vi "rsscope_core_global.vi"() -> ()   [LabVIEW 2018] (continued)
of the modulation signal for the FM modulation types.\n\nAvailable Repeated Capabilities:\nWaveformGenerator: WG1, WG2\r\n\nRemote-control command(s):\nWGENerator<m>:MODulation:FM[:FUNCtion]"}, {"Level"=5, "Class Only"=FALSE, "Identifier"="RSSCOPE_ATTR_WAVEFORM_GENERATOR_FM_MODULATION_FREQUENCY", "Descriptive Name"="Waveform Generator FM Modulation Frequency", "Data Type"=1, "Command"="WGEN{WaveformGenerator}:MOD:FM:FREQ", "Access"=2, "Range Table"="RsScope_rngWaveformGeneratorModulationFrequency", "Read Callback"="", "Write Callback"="", "Supported Models"="", "Instrument Options"="B6", "Flags"=0, "Help"="Sets the frequency of the modulation waveform for frequency modulation.\n\nAvailable Repeated Capabilities:\nWaveformGenerator: WG1, WG2\r\n\nRemote-control command(s):\nWGENerator<m>:MODulation:FM:FREQuency"}, {"Level"=5, "Class Only"=FALSE, "Identifier"="RSSCOPE_ATTR_WAVEFORM_GENERATOR_FM_MODULATION_FREQUENCY_DEVIATION", "Descriptive Name"="Waveform Generator FM Modulation Frequency Deviation", "Data Type"=1, "Command"="WGEN{WaveformGenerator}:MOD:FM:DEV", "Access"=2, "Range Table"="RsScope_rngWaveformGeneratorFMModulationFrequencyDeviation", "Read Callback"="", "Write Callback"="", "Supported Models"="", "Instrument Options"="B6", "Flags"=0, "Help"="Sets the frequency deviation, the maximum difference between and FM modulated signal and the carrier signal.\n\nAvailable Repeated Capabilities:\nWaveformGenerator: WG1, WG2\r\n\nRemote-control command(s):\nWGENerator<m>:MODulation:FM:DEViation"}, {"Level"=5, "Class Only"=FALSE, "Identifier"="RSSCOPE_ATTR_WAVEFORM_GENERATOR_FM_MODULATION_DUTY_CYCLE", "Descriptive Name"="Waveform Generator FM Modulation Duty Cycle", "Data Type"=1, "Command"="WGEN{WaveformGenerator}:MOD:FM:DCYC", "Access"=2, "Range Table"="RsScope_rngWaveformGeneratorModulationDutyCycle", "Read Callback"="", "Write Callback"="", "Supported Models"="", "Instrument Options"="B6", "Flags"=0, "Help"="Sets the duty cycle of a square waveform for frequency modulation.\n\nAvailable Repeated Capabilities:\nWaveformGenerator: WG1, WG2\r\n\nRemote-control command(s):\nWGENerator<m>:MODulation:FM:DCYCle"}, {"Level"=5, "Class Only"=FALSE, "Identifier"="RSSCOPE_ATTR_WAVEFORM_GENERATOR_FM_MODULATION_SYMMETRY", "Descriptive Name"="Waveform Generator FM Modulation Symmetry", "Data Type"=1, "Command"="WGEN{WaveformGenerator}:MOD:FM:SYMM", "Access"=2, "Range Table"="RsScope_rngPercent", "Read Callback"="", "Write Callback"="", "Supported Models"="", "Instrument Options"="B6", "Flags"=0, "Help"="Sets the symmetry, the percentage of time the ramp modulation waveform is rising, for frequency modulation.\n\nAvailable Repeated Capabilities:\nWaveformGenerator: WG1, WG2\r\n\nRemote-control command(s):\nWGENerator<m>:MODulation:FM:SYMMetry"}, {"Level"=4, "Class Only"=TRUE, "Identifier"="", "Descriptive Name"="PWM", "Data Type"=0, "Command"="", "Access"=0, "Range Table"="", "Read Callback"="", "Write Callback"="", "Supported Models"="", "Instrument Options"="", "Flags"=0, "Help"="For pulse width modulation (PWM), the time for which the signal is in a high state is varied according to the modulation signal."}, {"Level"=5, "Class Only"=FALSE, "Identifier"="RSSCOPE_ATTR_WAVEFORM_GENERATOR_PWM_MODULATION_SIGNAL", "Descriptive Name"="Waveform Generator PWM Modulation Signal", "Data Type"=0, "Command"="WGEN{WaveformGenerator}:MOD:PWM", "Access"=2, "Range Table"="RsScope_rngWaveformGeneratorModulationSignal", "Read Callback"="", "Write Callback"="", "Supported Models"="", "Instrument Options"="B6", "Flags"=0, "Help"="Selects the type of the modulation signal for the PWM modulation types.\n\nAvailable Repeated Capabilities:\nWaveformGenerator: WG1, WG2\r\n\nRemote-control command(s):\nWGENerator<m>:MODulation:PWM[:FUNCtion]"}, {"Level"=5, "Class Only"=FALSE, "Identifier"="RSSCOPE_ATTR_WAVEFORM_GENERATOR_PWM_MODULATION_FREQUENCY", "Descriptive Name"="Waveform Generator PWM Modulation Frequency", "Data Type"=1, "Command"="WGEN{WaveformGenerator}:MOD:PWM:FREQ", "Access"=2, "Range Table"="RsScope_rngWaveformGeneratorModulationFrequency", "Read Callback"="", "Write Callback"="", "Supported Models"="", "Instrument Options"="B6", "Flags"=0, "Help"="Sets the type of the modulation signal for the pulse width modulation.\n\nAvailable Repeated Capabilities:\nWaveformGenerator: WG1, WG2\r\n\nRemote-control command(s):\nWGENerator<m>:MODulation:PWM:FREQuency"}, {"Level"=5, "Class Only"=FALSE, "Identifier"="RSSCOPE_ATTR_WAVEFORM_GENERATOR_PWM_MODULATION_DEPTH", "Descriptive Name"="Waveform Generator PWM Modulation Depth", "Data Type"=1, "Command"="WGEN{WaveformGenerator}:MOD:PWM:DEPT", "Access"=2, "Range Table"="RsScope_rngPercent", "Read Callback"="", "Write Callback"="", "Supported Models"="", "Instrument Options"="B6", "Flags"=0, "Help"="Sets the modulation depth for pulse width modulation.\n\nAvailable Repeated Capabilities:\nWaveformGenerator: WG1, WG2\r\n\nRemote-control command(s):\nWGENerator<m>:MODulation:PWM:DEPTh"}, {"Level"=5, "Class Only"=FALSE, "Identifier"="RSSCOPE_ATTR_WAVEFORM_GENERATOR_PWM_MODULATION_DUTY_CYCLE", "Descriptive Name"="Waveform Generator PWM Modulation Duty Cycle", "Data Type"=1, "Command"="WGEN{WaveformGenerator}:MOD:PWM:DCYC", "Access"=2, "Range Table"="RsScope_rngWaveformGeneratorModulationDutyCycle", "Read Callback"="", "Write Callback"="", "Supported Models"="", "Instrument Options"="B6", "Flags"=0, "Help"="Sets the duty cycle of a square waveform for pulse width modulation.\n\nAvailable Repeated Capabilities:\nWaveformGenerator: WG1, WG2\r\n\nRemote-control command(s):\nWGENerator<m>:MODulation:PWM:DCYCle"}, {"Level"=5, "Class Only"=FALSE, "Identifier"="RSSCOPE_ATTR_WAVEFORM_GENERATOR_PWM_MODULATION_SYMMETRY", "Descriptive Name"="Waveform Generator PWM Modulation Symmetry", "Data Type"=1, "Command"="WGEN{WaveformGenerator}:MOD:PWM:SYMM", "Access"=2, "Range Table"="RsScope_rngPercent", "Read Callback"="", "Write Callback"="", "Supported Models"="", "Instrument Options"="B6", "Flags"=0, "Help"="Sets the symmetry, the percentage of time the ramp modulation waveform is rising, for pulse width modulation.\n\nAvailable Repeated Capabilities:\nWaveformGenerator: WG1, WG2\r\n\nRemote-control command(s):\nWGENerator<m>:MODulation:PWM:SYMMetry"}, {"Level"=4, "Class Only"=TRUE, "Identifier"="", "Descriptive Name"="FSK", "Data Type"=0, "Command"="", "Access"=0, "Range Table"="", "Read Callback"="", "Write Callback"="", "Supported Models"="", "Instrument Options"="", "Flags"=0, "Help"="For frequency shift keying (FSK) modulation, the signal switches between Frequency 1 and Frequency 2 at a Hop rate."}, {"Level"=5, "Class Only"=FALSE, "Identifier"="RSSCOPE_ATTR_WAVEFORM_GENERATOR_FSK_MODULATION_FREQUENCY_1", "Descriptive Name"="Waveform Generator FSK Modulation Frequency 1", "Data Type"=1, "Command"="WGEN{WaveformGenerator}:MOD:FSK:FONE", "Access"=2, "Range Table"="RsScope_rngWaveformGeneratorFrequency", "Read Callback"="", "Write Callback"="", "Supported Models"="", "Instrument Options"="B6", "Flags"=0, "Help"="Sets the frequency of the carrier waveform.\n\nAvailable Repeated Capabilities:\nWaveformGenerator: WG1, WG2\r\n\nRemote-control command(s):\nWGENerator<m>:MODulation:FSK:FONE"}, {"Level"=5, "Class Only"=FALSE, "Identifier"="RSSCOPE_ATTR_WAVEFORM_GENERATOR_FSK_MODULATION_FREQUENCY_2", "Descriptive Name"="Waveform Generator FSK Modulation Frequency 2", "Data Type"=1, "Command"="WGEN{WaveformGenerator}:MOD:FSK:FTWO", "Access"=2, "Range Table"="RsScope_rngWaveformGeneratorFrequency", "Read Callback"="", "Write Callback"="", "Supported Models"="", "Instrument Options"="B6", "Flags"=0, "Help"="Sets the frequency of the modulated waveform.\n\nAvailable Repeated Capabilities:\nWaveformGenerator: WG1, WG2\r\n\nRemote-control command(s):\nWGENerator<m>:MODulation:FSK:FTWO"}, {"Level"=5, "Class Only"=FALSE, "Identifier"="RSSCOPE_ATTR_WAVEFORM_GENERATOR_FSK_MODULATION_HOP_RATE", "Descriptive Name"="Waveform Generator FSK Modulation Hop Rate", "Data Type"=1, "Command"="WGEN{WaveformGenerator}:MOD:FSK", "Access"=2, "Range Table"="RsScope_rngWaveformGeneratorFSKModulationHopRate", "Read Callback"="", "Write Callback"="", "Supported Models"="", "Instrument Options"="B6", "Flags"=0, "Help"="Sets the hop rate, the time before a switch from the carrier frequency and the modulation frequency.\n\nAvailable Repeated Capabilities:\nWaveformGenerator: WG1, WG2\r\n\nRemote-control command(s):\nWGENerator<m>:MODulation:FSK[:RATE]"}, {"Level"=3, "Class Only"=TRUE, "Identifier"="", "Descriptive Name"="Sweep", "Data Type"=0, "Command"="", "Access"=0, "Range Table"="", "Read Callback"="", "Write Callback"="", "Supported Models"="", "Instrument Options"="", "Flags"=0, "Help"="In the sweep mode, the R&S RTO generates a signal whose frequency gradually changes from the Start frequency to the Stop freuqency for a certain Sweep time."}, {"Level"=4, "Class Only"=FALSE, "Identifier"="RSSCOPE_ATTR_WAVEFORM_GENERATOR_SWEEP_START_FREQUENCY", "Descriptive Name"="Waveform Generator Sweep Start Frequency", "Data Type"=1, "Command"="WGEN{WaveformGenerator}:SWE:FST", "Access"=2, "Range Table"="RsScope_rngWaveformGeneratorFrequency", "Read Callback"="", "Write Callback"="", "Supported Models"="", "Instrument Options"="B6", "Flags"=0, "Help"="Sets the start frequency of the sweep range.\n\nAvailable Repeated Capabilities:\nWaveformGenerator: WG1, WG2\r\n\nRemote-control command(s):\nWGENerator<m>:SWEep:FSTart"}, {"Level"=4, "Class Only"=FALSE, "Identifier"="RSSCOPE_ATTR_WAVEFORM_GENERATOR_SWEEP_STOP_FREQUENCY", "Descriptive Name"="Waveform Generator Sweep Stop Frequency", "Data Type"=1, "Command"="WGEN{WaveformGenerator}:SWE", "Access"=2, "Range Table"="RsScope_rngWaveformGeneratorFrequency", "Read Callback"="", "Write Callback"="", "Supported Models"="", "Instrument Options"="B6", "Flags"=0, "Help"="Sets the stop frequency of the sweep range.\n\nAvailable Repeated Capabilities:\nWaveformGenerator: WG1, WG2\r\n\nRemote-control command(s):\nWGENerator<m>:SWEep[:FEND]"}, {"Level"=4, "Class Only"=FALSE, "Identifier"="RSSCOPE_ATTR_WAVEFORM_GENERATOR_SWEEP_TIME", "Descriptive Name"="Waveform Generator Sweep Time", "Data Type"=1, "Command"="WGEN{WaveformGenerator}:SWE:TIME", "Access"=2, "Range Table"="RsScope_rngWaveformGeneratorSweepTime", "Read Callback"="", "Write Callback"="", "Supported Models"="", "Instrument Options"="B6", "Flags"=0, "Help"="Sets the duration of the sweep.\n\nAvailable Repeated Capabilities:\nWaveformGenerator: WG1, WG2\r\n\nRemote-control command(s):\nWGENerator<m>:SWEep:TIME"}, {"Level"=3, "Class Only"=TRUE, "Identifier"="", "Descriptive Name"="Arbitrary", "Data Type"=0, "Command"="", "Access"=0, "Range Table"="", "Read Callback"="", "Write Callback"="", "Supported Models"="", "Instrument Options"="", "Flags"=0, "Help"="The arbitrary waveform generator allows you to output a user-defined waveform for testing your devices. You can output a waveform from a file or from the current R&S RTO reference curve format. Files in *.csv and *.bin formats are supported. This files must follow a defined structure."}, {"Level"=4, "Class Only"=FALSE, "Identifier"="RSSCOPE_ATTR_WAVEFORM_GENERATOR_ARBITRARY_SOURCE", "Descriptive Name"="Waveform Generator Arbitrary Source", "Data Type"=0, "Command"="WGEN{WaveformGenerator}:ARBG", "Access"=2, "Range Table"="RsScope_rngWaveformGeneratorArbitrarySource", "Read Callback"="", "Write Callback"="", "Supported Models"="", "Instrument Options"="B6", "Flags"=0, "Help"="Selects the arbitrary waveform source. You can load an existing file or load the current oscilloscope waveform.\n\nAvailable Repeated Capabilities:\nWaveformGenerator: WG1, WG2\r\n\nRemote-control command(s):\nWGENerator<m>:ARBGen[:SOURce]"}, {"Level"=4, "Class Only"=FALSE, "Identifier"="RSSCOPE_ATTR_WAVEFORM_GENERATOR_ARBITRARY_RUN_MODE", "Descriptive Name"="Waveform Generator Arbitrary Run Mode", "Data Type"=0, "Command"="WGEN{WaveformGenerator}:ARBG:RUNM", "Access"=2, "Range Table"="RsScope_rngWaveformGeneratorRunMode", "Read Callback"="", "Write Callback"="", "Supported Models"="", "Instrument Options"="B6", "Flags"=0, "Help"="Sets the duration for which the signal of the arbitrary generator will be output after the trigger event.\n\nAvailable Repeated Capabilities:\nWaveformGenerator: WG1, WG2\r\n\nRemote-control command(s):\nWGENerator<m>:ARBGen:RUNMode"}, {"Level"=4, "Class Only"=FALSE, "Identifier"="RSSCOPE_ATTR_WAVEFORM_GENERATOR_ARBITRARY_RUN_SINGLE", "Descriptive Name"="Waveform Generator Arbitrary Run Single", "Data Type"=4, "Command"="WGEN{WaveformGenerator}:ARBG:RUNS", "Access"=1, "Range Table"="", "Read Callback"="", "Write Callback"="", "Supported Models"="", "Instrument Options"="", "Flags"=0, "Help"="Executes a single period of the arbitrary signal generator.\n\nAvailable Repeated Capabilities:\nWaveformGenerator: WG1, WG2\r\n\nRemote-control command(s):\nWGENerator<m>:ARBGen:RUNSingle"}, {"Level"=4, "Class Only"=FALSE, "Identifier"="RSSCOPE_ATTR_WAVEFORM_GENERATOR_ARBITRARY_SAMPLE_RATE", "Descriptive Name"="Waveform Generator Arbitrary Sample Rate", "Data Type"=0, "Command"="WGEN{WaveformGenerator}:ARBG:SRAT", "Access"=2, "Range Table"="RsScope_rngWaveformGeneratorArbitrarySampleRate", "Read Callback"="", "Write Callback"="", "Supported Models"="", "Instrument Options"="B6", "Flags"=0, "Help"="Sets the sample rate for the arbitrary waveform.\n\nAvailable Repeated Capabilities:\nWaveformGenerator: WG1, WG2\r\n\nRemote-control command(s):\nWGENerator<m>:ARBGen:SRATe"}, {"Level"=4, "Class Only"=FALSE, "Identifier"="RSSCOPE_ATTR_WAVEFORM_GENERATOR_ARBITRARY_SAMPLES", "Descriptive Name"="Waveform Generator Arbitrary Samples", "Data Type"=0, "Command"="WGEN{WaveformGenerator}:ARBG:SAMP?", "Access"=0, "Range Table"="", "Read Callback"="", "Write Callback"="", "Supported Models"="", "Instrument Options"="B6", "Flags"=0, "Help"="Displays the number of samples in the loaded waveform.\n\nAvailable Repeated Capabilities:\nWaveformGenerator: WG1, WG2\r\n\nRemote-control command(s):\nWGENerator<m>:ARBGen:SAMPles?"}, {"Level"=4, "Class Only"=TRUE, "Identifier"="", "Descriptive Name"="Saved Waveform", "Data Type"=0, "Command"="", "Access"=0, "Range Table"="", "Read Callback"="", "Write Callback"="", "Supported Models"="", "Instrument Options"="", "Flags"=0, "Help"="Configures arbitrary saved waveform."}, {"Level"=5, "Class Only"=FALSE, "Identifier"="RSSCOPE_ATTR_WAVEFORM_GENERATOR_ARBITRARY_FILE_NAME", "Descriptive Name"="Waveform Generator Arbitrary File Name", "Data Type"=2, "Command"="WGEN{WaveformGenerator}:ARBG:NAME", "Access"=2, "Range Table"="", "Read Callback"="", "Write Callback"="", "Supported Models"="", "Instrument Options"="B6", "Flags"=0, "Help"="Sets the file path and the file for an arbitrary waveform.\n\nAvailable Repeated Capabilities:\nWaveformGenerator: WG1, WG2\r\n\nRemote-control command(s):\nWGENerator<m>:ARBGen:NAME"}, {"Level"=5, "Class Only"=FALSE, "Identifier"="RSSCOPE_ATTR_WAVEFORM_GENERATOR_ARBITRARY_OPEN_FILE", "Descriptive Name"="Waveform Generator Arbitrary Open File", "Data Type"=4, "Command"="WGEN{WaveformGenerator}:ARBG:OPEN", "Access"=1, "Range Table"="", "Read Callback"="", "Write Callback"="", "Supported Models"="", "Instrument Options"="B6", "Flags"=0, "Help"="Loads the arbitrary waveform.\n\nAvailable Repeated Capabilities:\nWaveformGenerator: WG1, WG2\r\n\nRemote-control command(s):\nWGENerator<m>:ARBGen:OPEN"}, {"Level"=5, "Class Only"=FALSE, "Identifier"="RSSCOPE_ATTR_WAVEFORM_GENERATOR_ARBITRARY_MULTICHANNEL_FILE_NAME", "Descriptive Name"="Waveform Generator Arbitrary Multichannel File Name", "Data Type"=2, "Command"="WGEN{WaveformGenerator}:ARBG:MULT:NAME", "Access"=2, "Range Table"="", "Read Callback"="", "Write Callback"="", "Supported Models"="", "Instrument Options"="B6", "Flags"=0, "Help"="Defines the path and the multichannel arbitrary waveform file to be imported.\n\nAvailable Repeated Capabilities:\nWaveformGenerator: WG1, WG2\r\n\nRemote-control command(s):\nWGENerator<m>:ARBGen:MULTichannel:NAME"}, {"Level"=5, "Class Only"=FALSE, "Identifier"="RSSCOPE_ATTR_WAVEFORM_GENERATOR_ARBITRARY_MULTICHANNEL_OPEN_FILE", "Descriptive Name"="Waveform Generator Arbitrary Multichannel Open File", "Data Type"=4, "Command"="WGEN{WaveformGenerator}:ARBG:MULT:OPEN", "Access"=1, "Range Table"="", "Read Callback"="", "Write Callback"="", "Supported Models"="", "Instrument Options"="B6", "Flags"=0, "Help"="Loads the arbitrary waveform.\n\nAvailable Repeated Capabilities:\nWaveformGenerator: WG1, WG2\r\n\nRemote-control command(s):\nWGENerator<m>:ARBGen:MULTichannel:OPEN"}, {"Level"=5, "Class Only"=FALSE, "Identifier"="RSSCOPE_ATTR_WAVEFORM_GENERATOR_ARBITRARY_MULTICHANNEL_WAVEFORM", "Descriptive Name"="Waveform Generator Arbitrary Multichannel Waveform", "Data Type"=0, "Command"="WGEN{WaveformGenerator}:ARBG:MULT:IMP", "Access"=2, "Range Table"="RsScope_rngWaveformGeneratorArbitraryMultichannelWaveform", "Read Callback"="", "Write Callback"="", "Supported Models"="", "Instrument Options"="B6", "Flags"=0, "Help"="Assigns a waveform from the multichannel file to the arbitrary waveform generator.\n\nAvailable Repeated Capabilities:\nWaveformGenerator: WG1, WG2\r\n\nRemote-control command(s):\nWGENerator<m>:ARBGen:MULTichannel:IMPort"}, {"Level"=4, "Class Only"=TRUE, "Identifier"="", "Descriptive Name"="Scope Waveform", "Data Type"=0, "Command"="", "Access"=0, "Range Table"="", "Read Callback"="", "Write Callback"="", "Supported Models"="", "Instrument Options"="", "Flags"=0, "Help"="Configures arbitrary scope waveform."}, {"Level"=5, "Class Only"=FALSE, "Identifier"="RSSCOPE_ATTR_WAVEFORM_GENERATOR_ARBITRARY_SCOPE_SOURCE", "Descriptive Name"="Waveform Generator Arbitrary Scope Source", "Data Type"=0, "Command"="WGEN{WaveformGenerator}:ARBG:SEL", "Access"=2, "Range Table"="RsScope_rngWaveformGeneratorArbitraryScopeSource", "Read Callback"="", "Write Callback"="", "Supported Models"="", "Instrument Options"="B6", "Flags"=0, "Help"="Selects the oscilloscope source, from which the arbitrary signal is loaded.\n\nAvailable Repeated Capabilities:\nWaveformGenerator: WG1, WG2\r\n\nRemote-control command(s):\nWGENerator<m>:ARBGen:SELect"}, {"Level"=5, "Class Only"=FALSE, "Identifier"="RSSCOPE_ATTR_WAVEFORM_GENERATOR_ARBITRARY_SCOPE_OPEN", "Descriptive Name"="Waveform Generator Arbitrary Scope Open", "Data Type"=4, "Command"="WGEN{WaveformGenerator}:ARBG:COPY", "Access"=1, "Range Table"="", "Read Callback"="", "Write Callback"="", "Supported Models"="", "Instrument Options"="B6", "Flags"=0, "Help"="Loads the waveform from the selected signal source.\n\nAvailable Repeated Capabilities:\nWaveformGenerator: WG1, WG2\r\n\nRemote-control command(s):\nWGENerator<m>:ARBGen:COPY"}, {"Level"=3, "Class Only"=TRUE, "Identifier"="", "Descriptive Name"="Output", "Data Type"=0, "Command"="", "Access"=0, "Range Table"="", "Read Callback"="", "Write Callback"="", "Supported Models"="", "Instrument Options"="", "Flags"=0, "Help"="Configures the output values of generator."}, {"Level"=4, "Class Only"=FALSE, "Identifier"="RSSCOPE_ATTR_WAVEFORM_GENERATOR_OUTPUT_AMPLITUDE", "Descriptive Name"="Waveform Generator Output Amplitude", "Data Type"=1, "Command"="WGEN{WaveformGenerator}:VOLT", "Access"=2, "Range Table"="RsScope_rngWaveformGeneratorOutputAmplitude", "Read Callback"="", "Write Callback"="", "Supported Models"="", "Instrument Options"="B6", "Flags"=0, "Help"="Sets the amplitude, peak to peak voltage, of the output waveform. This is defined as the voltage difference between the maximum and the minimum voltage levels.\n\nAvailable Repeated Capabilities:\nWaveformGenerator: WG1, WG2\r\n\nRemote-control command(s):\nWGENerator<m>:VOLTage[:VPP]"}, {"Level"=4, "Class Only"=FALSE, "Identifier"="RSSCOPE_ATTR_WAVEFORM_GENERATOR_OUTPUT_OFFSET", "Descriptive Name"="Waveform Generator Output Offset", "Data Type"=1, "Command"="WGEN{WaveformGenerator}:VOLT:OFFS", "Access"=2, "Range Table"="RsScope_rngWaveformGeneratorOutputOffset", "Read Callback"="", "Write Callback"="", "Supported Models"="", "Instrument Options"="B6", "Flags"=0, "Help"="Sets a voltage offset.\n\nAvailable Repeated Capabilities:\nWaveformGenerator: WG1, WG2\r\n\nRemote-control command(s):\nWGENerator<m>:VOLTage:OFFSet"}, {"Level"=4, "Class Only"=FALSE, "Identifier"="RSSCOPE_ATTR_WAVEFORM_GENERATOR_OUTPUT_HIGH_LEVEL", "Descriptive Name"="Waveform Generator Output High Level", "Data Type"=1, "Command"="WGEN{WaveformGenerator}:VOLT:HIGH", "Access"=2, "Range Table"="RsScope_rngWaveformGeneratorOutputHighLevel", "Read Callback"="", "Write Callback"="", "Supported Models"="", "Instrument Options"="B6", "Flags"=0, "Help"="Sets the high signal level of the output waveform.\n\nAvailable Repeated Capabilities:\nWaveformGenerator: WG1, WG2\r\n\nRemote-control command(s):\nWGENerator<m>:VOLTage:HIGH"}, {"Level"=4, "Class Only"=FALSE, "Identifier"="RSSCOPE_ATTR_WAVEFORM_GENERATOR_OUTPUT_LOW_LEVEL", "Descriptive Name"="Waveform Generator Output Low Level", "Data Type"=1, "Command"="WGEN{WaveformGenerator}:VOLT:LOW", "Access"=2, "Range Table"="RsScope_rngWaveformGeneratorOutputLowLevel", "Read Callback"="", "Write Callback"="", "Supported Models"="", "Instrument Options"="B6", "Flags"=0, "Help"="Sets the low signal level of the output waveform.\n\nAvailable Repeated Capabilities:\nWaveformGenerator: WG1, WG2\r\n\nRemote-control command(s):\nWGENerator<m>:VOLTage:LOW"}, {"Level"=4, "Class Only"=FALSE, "Identifier"="RSSCOPE_ATTR_WAVEFORM_GENERATOR_OUTPUT_INVERSION", "Descriptive Name"="Waveform Generator Output Inversion", "Data Type"=3, "Command"="WGEN{WaveformGenerator}:VOLT:INV", "Access"=2, "Range Table"="", "Read Callback"="", "Write Callback"="", "Supported Models"="", "Instrument Options"="B6", "Flags"=0, "Help"="Inverts the waveform at the offset level.\n\nAvailable Repeated Capabilities:\nWaveformGenerator: WG1, WG2\r\n\nRemote-control command(s):\nWGENerator<m>:VOLTage:INVersion"}, {"Level"=4, "Class Only"=FALSE, "Identifier"="RSSCOPE_ATTR_WAVEFORM_GENERATOR_OUTPUT_USER_LOAD", "Descriptive Name"="Waveform Generator Output User Load", "Data Type"=0, "Command"="WGEN{WaveformGenerator}:OUTP", "Access"=2, "Range Table"="RsScope_rngWaveformGeneratorLoad", "Read Callback"="", "Write Callback"="", "Supported Models"="", "Instrument Options"="B6", "Flags"=0, "Help"="Sets the load of the DUT at its connection.\n\nAvailable Repeated Capabilities:\nWaveformGenerator: WG1, WG2\r\n\nRemote-control command(s):\nWGENerator<m>:OUTPut[:LOAD]"}, {"Level"=4, "Class Only"=FALSE, "Identifier"="RSSCOPE_ATTR_WAVEFORM_GENERATOR_OUTPUT_DC_LEVEL", "Descriptive Name"="Waveform Generator Output DC Level", "Data Type"=1, "Command"="WGEN{WaveformGenerator}:VOLT:DCL", "Access"=2, "Range Table"="RsScope_rngWaveformGeneratorOutputDCLevel", "Read Callback"="", "Write Callback"="", "Supported Models"="", "Instrument Options"="B6", "Flags"=0, "Help"="Sets the DC level of the generated DC signal.\n\nAvailable Repeated Capabilities:\nWaveformGenerator: WG1, WG2\r\n\nRemote-control command(s):\nWGENerator<m>:VOLTage:DCLevel"}, {"Level"=3, "Class Only"=TRUE, "Identifier"="", "Descriptive Name"="Noise", "Data Type"=0, "Command"="", "Access"=0, "Range Table"="", "Read Callback"="", "Write Callback"="", "Supported Models"="", "Instrument Options"="", "Flags"=0, "Help"="Configures the noise of attributes."}, {"Level"=4, "Class Only"=FALSE, "Identifier"="RSSCOPE_ATTR_WAVEFORM_GENERATOR_ADD_NOISE", "Descriptive Name"="Waveform Generator Add Noise", "Data Type"=3, "Command"="WGEN{WaveformGenerator}:MOD:NOIS", "Access"=2, "Range Table"="", "Read Callback"="", "Write Callback"="", "Supported Models"="", "Instrument Options"="B6", "Flags"=0, "Help"="Enables the adding of noise to the waveform.\n\nAvailable Repeated Capabilities:\nWaveformGenerator: WG1, WG2\r\n\nRemote-control command(s):\nWGENerator<m>:MODulation:NOISe"}, {"Level"=4, "Class Only"=FALSE, "Identifier"="RSSCOPE_ATTR_WAVEFORM_GENERATOR_NOISE_LEVEL_PERCENT", "Descriptive Name"="Waveform Generator Noise Level Percent", "Data Type"=1, "Command"="WGEN{WaveformGenerator}:MOD:NLPC", "Access"=2, "Range Table"="RsScope_rngPercent", "Read Callback"="", "Write Callback"="", "Supported Models"="", "Instrument Options"="B6", "Flags"=0, "Help"="Sets the noise level in percentage of the amplitude.\n\nAvailable Repeated Capabilities:\nWaveformGenerator: WG1, WG2\r\n\nRemote-control command(s):\nWGENerator<m>:MODulation:NLPCent"}, {"Level"=4, "Class Only"=FALSE, "Identifier"="RSSCOPE_ATTR_WAVEFORM_GENERATOR_NOISE_ABSOLUTE_LEVEL", "Descriptive Name"="Waveform Generator Noise Absolute Level", "Data Type"=1, "Command"="WGEN{WaveformGenerator}:MOD:NLAB?", "Access"=0, "Range Table"="", "Read Callback"="", "Write Callback"="", "Supported Models"="", "Instrument Options"="B6", "Flags"=0, "Help"="Queries the level of the noise in volts.\n\nAvailable Repeated Capabilities:\nWaveformGenerator: WG1, WG2\r\n\nRemote-control command(s):\nWGENerator<m>:MODulation:NLABsolute?"}, {"Level"=4, "Class Only"=FALSE, "Identifier"="RSSCOPE_ATTR_WAVEFORM_GENERATOR_NOISE_DC_LEVEL", "Descriptive Name"="Waveform Generator Noise DC Level", "Data Type"=1, "Command"="WGEN{WaveformGenerator}:MOD:NDCL", "Access"=2, "Range Table"="RsScope_rngWaveformGeneratorNoiseDCLevel", "Read Callback"="", "Write Callback"="", "Supported Models"="", "Instrument Options"="B6", "Flags"=0, "Help"="Sets the DC noise level.\n\nAvailable Repeated Capabilities:\nWaveformGenerator: WG1, WG2\r\n\nRemote-control command(s):\nWGENerator<m>:MODulation:NDCLevel"}, {"Level"=3, "Class Only"=TRUE, "Identifier"="", "Descriptive Name"="Coupling", "Data Type"=0, "Command"="", "Access"=0, "Range Table"="", "Read Callback"="", "Write Callback"="", "Supported Models"="", "Instrument Options"="", "Flags"=0, "Help"="In the R&S RTO, you can couple certain settings of the available waveform generators.If one of the available coupling options is enabled for one of the generators, the values for all coupled parameters are automatically taken from the master generator."}, {"Level"=4, "Class Only"=FALSE, "Identifier"="RSSCOPE_ATTR_WAVEFORM_GENERATOR_COUPLING_ENABLE", "Descriptive Name"="Waveform Generator Coupling Enable", "Data Type"=3, "Command"="WGEN{WaveformGenerator}:COUP:STAT", "Access"=2, "Range Table"="", "Read Callback"="", "Write Callback"="", "Supported Models"="", "Instrument Options"="B6", "Flags"=0, "Help"="Enables the coupling of the generators, with the selected set of parameters: amplitude, frequency and noise.\n\nAvailable Repeated Capabilities:\nWaveformGenerator: WG1, WG2\r\n\nRemote-control command(s):\nWGENerator<m>:COUPling:STATe"}, {"Level"=4, "Class Only"=FALSE, "Identifier"="RSSCOPE_ATTR_WAVEFORM_GENERATOR_COUPLING_ALL", "Descriptive Name"="Waveform Generator Coupling All", "Data Type"=3, "Command"="WGEN{WaveformGenerator}:COUP:ALL", "Access"=2, "Range Table"="", "Read Callback"="", "Write Callback"="", "Supported Models"="", "Instrument Options"="B6", "Flags"=0, "Help"="Enables the coupling of all parameters of the generators, except of load and inversion.\n\nAvailable Repeated Capabilities:\nWaveformGenerator: WG1, WG2\r\n\nRemote-control command(s):\nWGENerator<m>:COUPling:ALL"}, {"Level"=4, "Class Only"=FALSE, "Identifier"="RSSCOPE_ATTR_WAVEFORM_GENERATOR_COUPLING_OUTPUT", "Descriptive Name"="Waveform Generator Coupling Output", "Data Type"=3, "Command"="WGEN{WaveformGenerator}:COUP:OUTP", "Access"=2, "Range Table"="", "Read Callback"="", "Write Callback"="", "Supported Models"="", "Instrument Options"="", "Flags"=0, "Help"="Couples all parameters including output enable, but excluding inversion and load.\n\nAvailable Repeated Capabilities:\nWaveformGenerator: WG1, WG2\r\n\nRemote-control command(s):\nWGENerator<m>:COUPling:OUTPut"}, {"Level"=4, "Class Only"=FALSE, "Identifier"="RSSCOPE_ATTR_WAVEFORM_GENERATOR_COUPLING_NOISE", "Descriptive Name"="Waveform Generator Coupling Noise", "Data Type"=3, "Command"="WGEN{WaveformGenerator}:COUP:NOIS", "Access"=2, "Range Table"="", "Read Callback"="", "Write Callback"="", "Supported Models"="", "Instrument Options"="B6", "Flags"=0, "Help"="Couples all noise parameters of the generators.\n\nAvailable Repeated Capabilities:\nWaveformGenerator: WG1, WG2\r\n\nRemote-control command(s):\nWGENerator<m>:COUPling:NOISe"}, {"Level"=4, "Class Only"=FALSE, "Identifier"="RSSCOPE_ATTR_WAVEFORM_GENERATOR_COUPLING_ARBITRARY", "Descriptive Name"="Waveform Generator Coupling Arbitrary", "Data Type"=3, "Command"="WGEN{WaveformGenerator}:COUP:AWF", "Access"=2, "Range Table"="", "Read Callback"="", "Write Callback"="", "Supported Models"="", "Instrument Options"="B6", "Flags"=0, "Help"="Enables the coupling of the arbitrary waveform of the generators.\n\nAvailable Repeated Capabilities:\nWaveformGenerator: WG1, WG2\r\n\nRemote-control command(s):\nWGENerator<m>:COUPling:AWForm"}, {"Level"=4, "Class Only"=FALSE, "Identifier"="RSSCOPE_ATTR_WAVEFORM_GENERATOR_COUPLING_AMPLITUDE", "Descriptive Name"="Waveform Generator Coupling Amplitude", "Data Type"=3, "Command"="WGEN{WaveformGenerator}:COUP:AMP", "Access"=2, "Range Table"="", "Read Callback"="", "Write Callback"="", "Supported Models"="", "Instrument Options"="B6", "Flags"=0, "Help"="Enables the coupling of all amplitude parameters of the generators.\n\nAvailable Repeated Capabilities:\nWaveformGenerator: WG1, WG2\r\n\nRemote-control command(s):\nWGENerator<m>:COUPling:AMPLitude"}, {"Level"=4, "Class Only"=FALSE, "Identifier"="RSSCOPE_ATTR_WAVEFORM_GENERATOR_COUPLING_PHASE_SHIFT", "Descriptive Name"="Waveform Generator Coupling Phase Shift", "Data Type"=1, "Command"="WGEN{WaveformGenerator}:COUP:PHAS", "Access"=2, "Range Table"="RsScope_rngWaveformGeneratorCouplingPhaseShift", "Read Callback"="", "Write Callback"="", "Supported Models"="", "Instrument Options"="B6", "Flags"=0, "Help"="Sets the phase shift between the waveform of Gen1 and Gen2 when the frequency parameters of the two waveforms are coupled.\n\nAvailable Repeated Capabilities:\nWaveformGenerator: WG1, WG2\r\n\nRemote-control command(s):\nWGENerator<m>:COUPling:PHASeshift"}, {"Level"=4, "Class Only"=FALSE, "Identifier"="RSSCOPE_ATTR_WAVEFORM_GENERATOR_COUPLING_FREQUENCY", "Descriptive Name"="Waveform Generator Coupling Frequency", "Data Type"=3, "Command"="WGEN{WaveformGenerator}:COUP", "Access"=2, "Range Table"="", "Read Callback"="", "Write Callback"="", "Supported Models"="", "Instrument Options"="B6", "Flags"=0, "Help"="Enables the coupling of all frequency parameters of the generators.\n\nAvailable Repeated Capabilities:\nWaveformGenerator: WG1, WG2\r\n\nRemote-control command(s):\nWGENerator<m>:COUPling[:FREQuency]"}, {"Level"=2, "Class Only"=TRUE, "Identifier"="", "Descriptive Name"="Pattern Generator", "Data Type"=0, "Command"="", "Access"=0, "Range Table"="", "Read Callback"="", "Write Callback"="", "Supported Models"="", "Instrument Options"="", "Flags"=0, "Help"="Includes an integrated pattern generator which can generate patterns during testing."}, {"Level"=3, "Class Only"=FALSE, "Identifier"="RSSCOPE_ATTR_PATTERN_GENERATOR_ENABLE", "Descriptive Name"="Pattern Generator Enable", "Data Type"=3, "Command"="PGEN:ENAB", "Access"=2, "Range Table"="", "Read Callback"="", "Write Callback"="", "Supported Models"="", "Instrument Options"="B6", "Flags"=0, "Help"="Enables the pattern generator and outputs the waveform.\n\nAvailable Repeated Capabilities:\nNone\n\nRemote-control command(s):\nPGENerator:ENABle"}, {"Level"=3, "Class Only"=FALSE, "Identifier"="RSSCOPE_ATTR_PATTERN_GENERATOR_PRESET", "Descriptive Name"="Pattern Generator Preset", "Data Type"=4, "Command"="PGEN:PRES", "Access"=1, "Range Table"="", "Read Callback"="", "Write Callback"="", "Supported Models"="", "Instrument Options"="B6", "Flags"=0, "Help"="Sets the parameters of the waveform generator to their default values.\n\nAvailable Repeated Capabilities:\nNone\n\nRemote-control command(s):\nPGENerator:PRESet"}, {"Level"=3, "Class Only"=FALSE, "Identifier"="RSSCOPE_ATTR_PATTERN_GENERATOR_RUN_MODE", "Descriptive Name"="Pattern Generator Run Mode", "Data Type"=0, "Command"="PGEN:RUNM", "Access"=2, "Range Table"="RsScope_rngWaveformGeneratorRunMode", "Read Callback"="", "Write Callback"="", "Supported Models"="", "Instrument Options"="B6", "Flags"=0, "Help"="Sets the duration for which the signal of the pattern generator will be output after the trigger event.\n\nAvailable Repeated Capabilities:\nNone\n\nRemote-control command(s):\nPGENerator:RUNMode"}, {"Level"=3, "Class Only"=FALSE, "Identifier"="RSSCOPE_ATTR_PATTERN_GENERATOR_RUN_SINGLE", "Descriptive Name"="Pattern Generator Run Single", "Data Type"=4, "Command"="PGEN:RUNS", "Access"=1, "Range Table"="", "Read Callback"="", "Write Callback"="", "Supported Models"="", "Instrument Options"="", "Flags"=0, "Help"="Executes a single period of the pattern generator, for PGENerator:RUNMode SINGle.\n\nAvailable Repeated Capabilities:\nNone\n\nRemote-control command(s):\nPGENerator:RUNSingle"}, {"Level"=3, "Class Only"=FALSE, "Identifier"="RSSCOPE_ATTR_PATTERN_GENERATOR_BIT_RATE", "Descriptive Name"="Pattern Generator Bit Rate", "Data Type"=0, "Command"="PGEN:BITR", "Access"=2, "Range Table"="RsScope_rngPatternGeneratorBitRate", "Read Callback"="", "Write Callback"="", "Supported Models"="", "Instrument Options"="B6", "Flags"=0, "Help"="Sets the number of transmitted bits per second for the pattern generator.\n\nAvailable Repeated Capabilities:\nNone\n\nRemote-control command(s):\nPGENerator:BITRate"}, {"Level"=3, "Class Only"=FALSE, "Identifier"="RSSCOPE_ATTR_PATTERN_GENERATOR_HIGH_LEVEL", "Descriptive Name"="Pattern Generator High Level", "Data Type"=1, "Command"="PGEN:HLEV", "Access"=2, "Range Table"="RsScope_rngPatternGeneratorHighLevel", "Read Callback"="", "Write Callback"="", "Supported Models"="", "Instrument Options"="B6", "Flags"=0, "Help"="Sets the high level of the pattern generator signal.\n\nAvailable Repeated Capabilities:\nNone\n\nRemote-control command(s):\nPGENerator:HLEVel"}, {"Level"=3, "Class Only"=FALSE, "Identifier"="RSSCOPE_ATTR_PATTERN_GENERATOR_FILE_NAME", "Descriptive Name"="Pattern Generator File Name", "Data Type"=2, "Command"="PGEN:FILE", "Access"=2, "Range Table"="", "Read Callback"="", "Write Callback"="", "Supported Models"="", "Instrument Options"="B6", "Flags"=0, "Help"="Specifies a file path to open a pattern generator file.\n\nAvailable Repeated Capabilities:\nNone\n\nRemote-control command(s):\nPGENerator:FILE[:NAME]"}, {"Level"=3, "Class Only"=FALSE, "Identifier"="RSSCOPE_ATTR_PATTERN_GENERATOR_LOAD_PATTERN", "Descriptive Name"="Pattern Generator Load Pattern", "Data Type"=4, "Command"="PGEN:FILE:OPEN", "Access"=1, "Range Table"="", "Read Callback"="", "Write Callback"="", "Supported Models"="", "Instrument Options"="B6", "Flags"=0, "Help"="Loads the specified pattern file to the instrument.\n\nAvailable Repeated Capabilities:\nNone\n\nRemote-control command(s):\nPGENerator:FILE:OPEN"}, {"Level"=2, "Class Only"=TRUE, "Identifier"="", "Descriptive Name"="Synchronization", "Data Type"=0, "Command"="", "Access"=0, "Range Table"="", "Read Callback"="", "Write Callback"="", "Supported Models"="", "Instrument Options"="", "Flags"=0, "Help"="Sets which signals generated from the waveform generator are synchronized."}, {"Level"=3, "Class Only"=FALSE, "Identifier"="RSSCOPE_ATTR_GENERATOR_SYNCHRONIZATION", "Descriptive Name"="Generator Synchronization", "Data Type"=0, "Command"="GEN:SYNC", "Access"=2, "Range Table"="RsScope_rngGeneratorSynchronization", "Read Callback"="", "Write Callback"="", "Supported Models"="", "Instrument Options"="B6", "Flags"=0, "Help"="Sets which signals generated from the waveform generator are synchronized.\n\nAvailable Repeated Capabilities:\nNone\n\nRemote-control command(s):\nGENerator:SYNC[:COMBination]"}, {"Level"=2, "Class Only"=TRUE, "Identifier"="", "Descriptive Name"="DC Offset Alignment", "Data Type"=0, "Command"="", "Access"=0, "Range Table"="", "Read Callback"="", "Write Callback"="", "Supported Models"="", "Instrument Options"="", "Flags"=0, "Help"="Cofigures generator DC offset alignment."}, {"Level"=3, "Class Only"=FALSE, "Identifier"="RSSCOPE_ATTR_GENERATOR_START_ALIGNMENT", "Descriptive Name"="Generator Start Alignment", "Data Type"=4, "Command"="GEN:ALIG:DC", "Access"=1, "Range Table"="", "Read Callback"="", "Write Callback"="", "Supported Models"="", "Instrument Options"="B6", "Flags"=2, "Help"="Starts the alignment of the DC offset.\n\nAvailable Repeated Capabilities:\nNone\n\nRemote-control command(s):\nGENerator:ALIGnment:DC[:STARt]"}, {"Level"=3, "Class Only"=FALSE, "Identifier"="RSSCOPE_ATTR_GENERATOR_START_ALIGNMENT_WITH_OPC", "Descriptive Name"="Generator Start Alignment With OPC", "Data Type"=4, "Command"="GEN:ALIG:DC", "Access"=1, "Range Table"="", "Read Callback"="", "Write Callback"="", "Supported Models"="", "Instrument Options"="B6", "Flags"=1, "Help"="Starts the alignment of the DC offset.\n\nAvailable Repeated Capabilities:\nNone\n\nRemote-control command(s):\nGENerator:ALIGnment:DC[:STARt]"}, {"Level"=3, "Class Only"=FALSE, "Identifier"="RSSCOPE_ATTR_GENERATOR_ABORT_ALIGNMENT", "Descriptive Name"="Generator Abort Alignment", "Data Type"=4, "Command"="GEN:ALIG:DC:ABOR", "Access"=1, "Range Table"="", "Read Callback"="", "Write Callback"="", "Supported Models"="", "Instrument Options"="B6", "Flags"=0, "Help"="Aborts a DC offset alignment.\n\nAvailable Repeated Capabilities:\nNone\n\nRemote-control command(s):\nGENerator:ALIGnment:DC:ABORt"}, {"Level"=3, "Class Only"=FALSE, "Identifier"="RSSCOPE_ATTR_GENERATOR_ALIGNMENT_DATE", "Descriptive Name"="Generator Alignment Date", "Data Type"=2, "Command"="GEN:ALIG:DC:RES:DATE?", "Access"=0, "Range Table"="", "Read Callback"="", "Write Callback"="", "Supported Models"="", "Instrument Options"="B6", "Flags"=0, "Help"="Displays the date of the last performed DC offset alignment.\n\nAvailable Repeated Capabilities:\nNone\n\nRemote-control command(s):\nGENerator:ALIGnment:DC:RESult:DATE?"}, {"Level"=3, "Class Only"=FALSE, "Identifier"="RSSCOPE_ATTR_GENERATOR_ALIGNMENT_TIME", "Descriptive Name"="Generator Alignment Time", "Data Type"=2, "Command"="GEN:ALIG:DC:RES:TIME?", "Access"=0, "Range Table"="", "Read Callback"="", "Write Callback"="", "Supported Models"="", "Instrument Options"="B6", "Flags"=0, "Help"="Queries the time of the last performed DC offset alignment.\n\nAvailable Repeated Capabilities:\nNone\n\nRemote-control command(s):\nGENerator:ALIGnment:DC:RESult:TIME?"}, {"Level"=3, "Class Only"=FALSE, "Identifier"="RSSCOPE_ATTR_GENERATOR_ALIGNMENT_OVERALL_STATE", "Descriptive Name"="Generator Alignment Overall State", "Data Type"=0, "Command"="GEN:ALIG:DC:RES?", "Access"=0, "Range Table"="RsScope_rngGeneratorAlignmentOverallState", "Read Callback"="", "Write Callback"="", "Supported Models"="", "Instrument Options"="B6", "Flags"=0, "Help"="Queries the result of a DC offset alignment.\n\nAvailable Repeated Capabilities:\nNone\n\nRemote-control command(s):\nGENerator:ALIGnment:DC:RESult[:STATe]?"}, {"Level"=1, "Class Only"=TRUE, "Identifier"="", "Descriptive Name"="I/Q Software Interface", "Data Type"=0, "Command"="", "Access"=0, "Range Table"="", "Read Callback"="", "Write Callback"="", "Supported Models"="", "Instrument Options"="", "Flags"=0, "Help"="This class contains attributes to acquire modulated signals and attributes to output I/Q data for further analysis using other software, for example, MATLAB."}, {"Level"=2, "Class Only"=FALSE, "Identifier"="RSSCOPE_ATTR_IQ_MODE_STATE", "Descriptive Name"="IQ Mode State", "Data Type"=3, "Command"="IQ:STAT", "Access"=2, "Range Table"="", "Read Callback"="", "Write Callback"="", "Supported Models"="", "Instrument Options"="K11", "Flags"=0, "Help"="Activates the I/Q mode of the instrument.\n\nAvailable Repeated Capabilities:\nNone\n\nRemote-control command(s):\nIQ:STATe"}, {"Level"=2, "Class Only"=FALSE, "Identifier"="RSSCOPE_ATTR_IQ_INPUT_SAMPLE_RATE", "Descriptive Name"="IQ Input Sample Rate", "Data Type"=0, "Command"="IQ:INSR?", "Access"=0, 
